vi "Init.vi"(8 "error in (no error)":errorcluster, 10 "Response":string, 11 "Mock Instrument Interface In":refnum<class "Mock Instrument Interface.lvclass">) -> (0 "error out":errorcluster, 3 "Mock Instrument Interface Out":refnum<class "Mock Instrument Interface.lvclass">)   [LabVIEW 2020, in "Low Level PSU With Tests.lvlib" / "Mock Instrument Interface.lvclass"]
uses:
  Mock Instrument Interface.lvclass
  Mock Instrument Interface.lvclass/Mock Instrument Interface.ctl
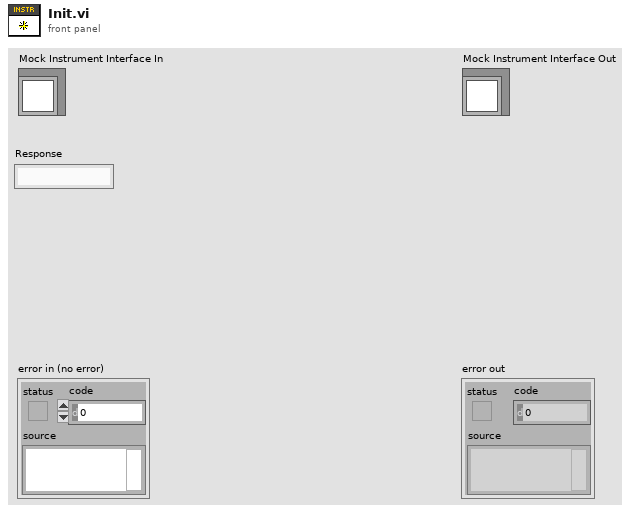
[diagram p1: front panel]
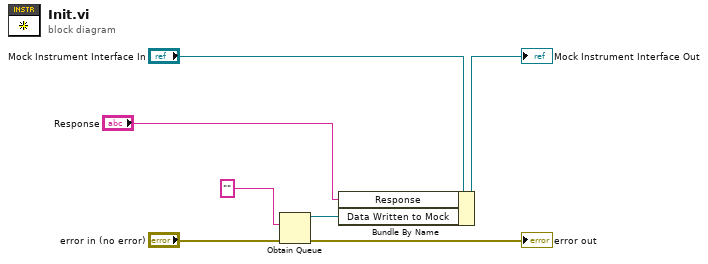
[diagram p0: block diagram]
diagram:
  n1 = Obtain Queue(element data type="", error in (no error)="error in (no error)") -> (queue out=w2:refnum<queue>, error out=→"error out":errorcluster)  [unwired: 3 in, 1 out]
  n2 = Bundle By Name(cluster="Mock Instrument Interface In", "Response"="Response", "Data Written to Mock"=w2) -> (→"Mock Instrument Interface Out":refnum<class "Mock Instrument Interface.lvclass">)
